vi "CreateDecoration.vi"(8 "error in":errorcluster, 11 "Decoration in":refnum<class "Decoration.lvclass">) -> (0 "error out":errorcluster, 3 "Decoration out":refnum<class "Decoration.lvclass">, 4 "decoration name":string, 6 "decoration":string)   [LabVIEW 2014, in "PythonConverter_GUI.lvclass"]
uses:
  PythonConverter_GUI.lvclass
  VI Interpreter/Classes/Decoration/Decoration.lvclass
  Parsing/Python Functions.lvlib
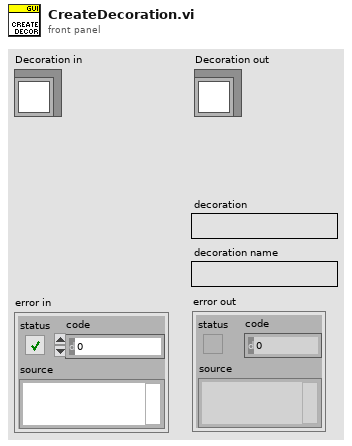
[diagram p1: front panel]
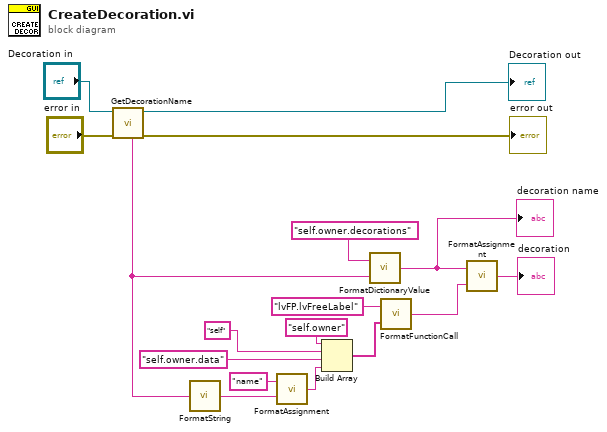
[diagram p0: block diagram]
diagram:
  n1 = call "GetDecorationName.vi"("error in"="error in", "Decoration in"="Decoration in") -> ("error out"=→"error out":errorcluster, "Decoration out"=→"Decoration out":refnum<class "Decoration.lvclass">, "name"=w8:string)  [unwired: 5 in]
  n2 = call "FormatString.vi"("value"=w8) -> ("python object"=w9:string)
  n3 = call "FormatAssignment.vi"("value"=w9, "name"="name") -> ("python assignment"=w10:string)
  n4 = Build Array("self.owner" ("String"), "self" ("name"), "self.owner.data" ("String"), w10) -> (w14:string[])
  n5 = call "FormatDictionaryValue.vi"("key"=w8, "dictionary"="self.owner.decorations") -> ("python object"=w4:string)
  "decoration name" <- w4
  n6 = call "FormatFunctionCall.vi"("parameters"=w14, "function"="lvFP.lvFreeLabel") -> ("python object"=w17:string)
  n7 = call "FormatAssignment.vi"("value"=w17, "name"=w4) -> ("python assignment"=→"decoration":string)
